vi "Teste tempo comunicacao.vi"() -> ()   [LabVIEW 2018]
panel:
  out "ms":u32
  out "response":string
  out "error out":errorcluster
  in  "instruction":string
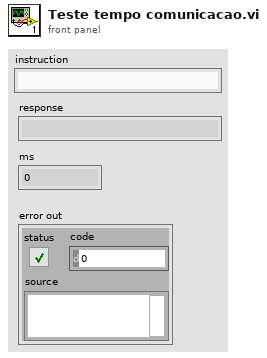
[diagram p1: front panel]
types:
  T1 = enum16{"Standard", "Buffered", "CRLF", "Immediate"}
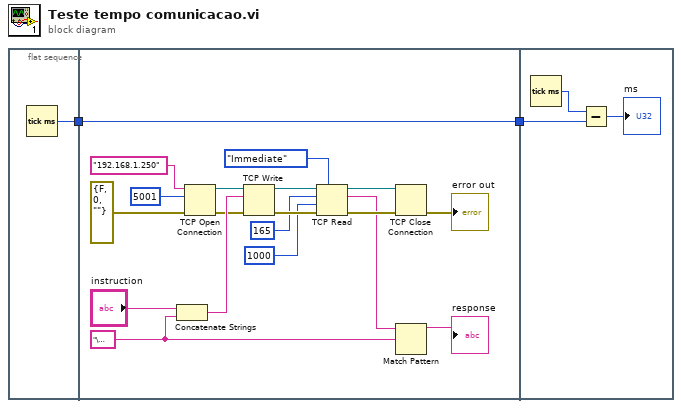
[diagram p0: block diagram]
diagram:
  n1 = flat-sequence {
    tunnel: [w3] -> w2
    tunnel: w2 -> [w4]
    tunnel: [w4] -> w1
    tunnel: w1 -> [w24]
    frame #0 {
      n2 = Tick Count (ms)() -> (millisecond timer value=w3:u32)
    }
    frame #1 {
      w7 = "\u0000" ("string")
      n3 = Concatenate Strings("instruction", w7) -> (w18:string)
      n4 = TCP Open Connection(address="192.168.1.250", remote port or service name=u16 5001, error in (no error)=errorcluster {"status"=FALSE, "code"=0, "source"=""}) -> (connection ID=w17:refnum<k5>, error out=w16:errorcluster)  [unwired: 2 in]
      n5 = TCP Write(connection ID=w17, data in=w18, error in (no error)=w16) -> (connection ID out=w15:refnum<k5>, error out=w14:errorcluster)  [unwired: 1 in, 1 out]
      n6 = TCP Read(connection ID=w15, bytes to read=165, error in (no error)=w14, 7:T1."Immediate" ("mode (standard)"), 9:1000 ("timeout ms (25000)")) -> (connection ID out=w10:refnum<k5>, data out=w6:string, error out=w9:errorcluster)
      n7 = TCP Close Connection(connection ID=w10, error in (no error)=w9) -> (error out=→"error out":errorcluster)  [unwired: 1 in, 1 out]
      n8 = Match Pattern(string=w6, regular expression=w7) -> (before substring=→"response":string)  [unwired: 1 in, 3 out]
    }
    frame #2 {
      n9 = Tick Count (ms)() -> (millisecond timer value=w25:u32)
      n10 = Subtract(x=w25, y=w24) -> (x-y=→"ms":u32)
    }
  }
